vi "QR二维码生成器.vi"(6 "保存按钮":bool, 7 "输入文本":string="殷培\n2013年9月5日\nemail:yin-pei@qq.com", 8 "掩模图形":u16(ring) items=["000", "001", "010", "011", "100", "101", "110", "111"], 9 "版本":u16(ring)=1 items=["1"=1, "2"=2, "3"=3, "4"=4, "5"=5, "6"=6, "7"=7, "8"=8, "9"=9, "10"=10, "11"=11, "12"=12, "13"=13, "14"=14, "15"=15, "16"=16, "17"=17, "18"=18, "19"=19, "20"=20, "21"=21, "22"=22, "23"=23, "24"=24, "25"=25, "26"=26, "27"=27, "28"=28, "29"=29, "30"=30, "31"=31, "32"=32, "33"=33, "34"=34, "35"=35, "36"=36, "37"=37, "38"=38, "39"=39, "40"=40], 10 "纠错等级":u16(ring)=2 items=["L(7%)", "M(15%)", "Q(25%)", "H(30%)"], 11 "自动？":enum16{"禁止自适应版本", "自适应版本"}(ring)=enum."自适应版本") -> (3 "new picture":picture caption="新图片")   [LabVIEW 2011]
uses:
  <vilib>/Utility/miscctls.llb/LVBoundsTypeDef.ctl
panel:
  in  "添加logo":bool
  in  "停止":bool
  in  "backcolor":u32(colorbox)=16777215
  in  "color":u32(colorbox)
  # "QR二维码生成器"
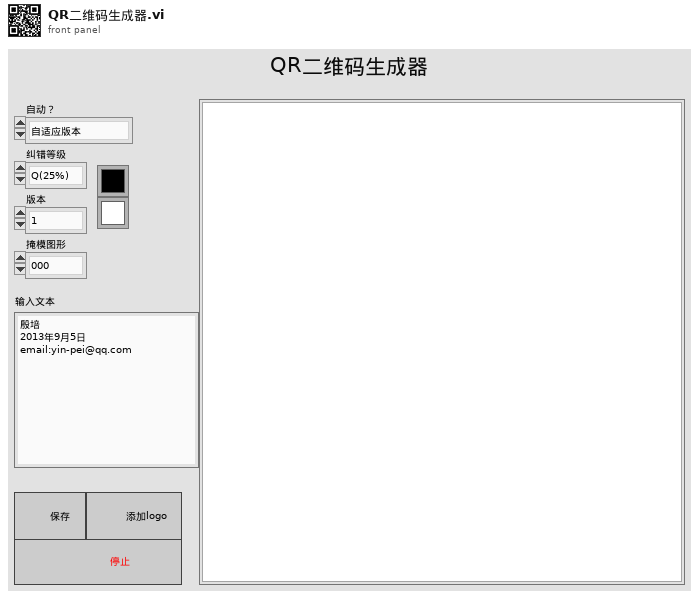
[diagram p1: front panel]
types:
  T1 = cluster{"left":i16, "top":i16, "right":i16, "bottom":i16}
  T2 = typedef "LVBoundsTypeDef.ctl" = cluster{"Width":u32, "Height":u32}
  T3 = typedef "imagedata.ctl" = cluster{"image type":i32, "image depth":i32, "image":u8[], "mask":u8[], "colors":u32[], "Rectangle":cluster{"left":i16, "top":i16, "right":i16, "bottom":i16}}
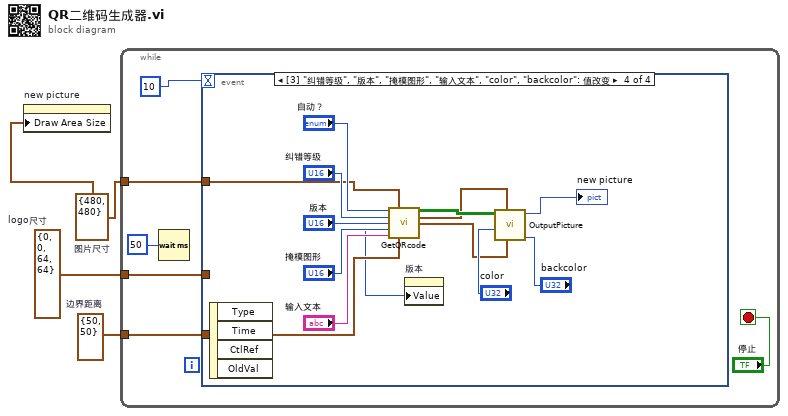
[diagram p0: block diagram]
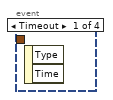
[diagram p2: hidden frame]
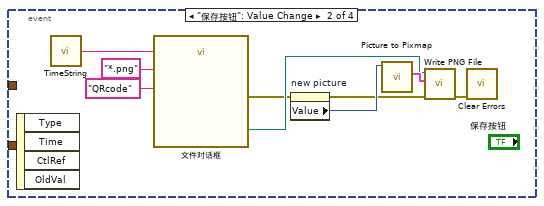
[diagram p3: hidden frame]
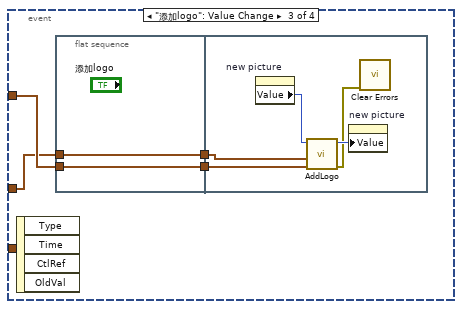
[diagram p4: hidden frame]
diagram:
  w1 = T1 {"left"=0, "top"=0, "right"=64, "bottom"=64}  # logo尺寸
  w2 = cluster{"x":i16, "y":i16} {"x"=50, "y"=50}  # 边界距离
  w3 = T2 {"Width"=480, "Height"=480}  # 图片尺寸
  n1 = property on="new picture" class="Pict"("Draw Area Size"=w3) -> ()  [unwired: 2 in, 2 out]
  n2 = while {
    tunnel: w3 -> [w6]
    tunnel: w2 -> [w5]
    tunnel: w1 -> [w4]
    stop <- "停止" stop-if-true
    n3 = Wait (ms)(milliseconds to wait=u32 50 ("等待时间（毫秒）")) -> ()  [unwired: 1 out]
    n4 = event shown="[3] \"纠错等级\", \"版本\", \"掩模图形\", \"输入文本\", \"color\", \"backcolor\": 值改变" {
      selector: _ -> [_ _ _ _]
      dyn-events: _ -> [_ _ _ _]
      timeout: 10 -> [_ _ _ _]
      tunnel: w6 -> [_ _ w22 w32]
      tunnel: w5 -> [_ _ _ w31]
      tunnel: w4 -> [_ _ w21 _]
      event Timeout {
        n5 = event-data() -> ()  [unwired: 1 in, 2 out]
      }
      event "保存按钮": Value Change {
        n6 = event-data() -> ()  [unwired: 1 in, 4 out]
        n7 = call "TimeString.vi"() -> ("时间字符串"=w12:string)
        n8 = call "文件对话框"("default name"=w12, "pattern (all files)"="*.png", "pattern label"="QRcode") -> ("selected path"=w14:path, "error out"=w13:errorcluster)  [unwired: 9 in, 2 out]
        n9 = property on="new picture" class="Pict"(error in=w13) -> (error out=w15:errorcluster, "Value"=w18:picture)  [unwired: 1 in, 1 out]
        n10 = call <vilib>:"Picture to Pixmap.vi"("picture"=w18) -> ("image data"=w17:T3)  [unwired: 9 in, 1 out]
        n11 = call <vilib>:"Write PNG File.vi"("error in (no error)"=w15, "image data"=w17, "path to PNG file"=w14) -> ("error out"=w16:errorcluster)  [unwired: 7 in, 1 out]
        n12 = call <vilib>:"Clear Errors.vi"("error in (no error)"=w16) -> ()  [unwired: 6 in, 1 out]
      }
      event "添加logo": Value Change {
        n13 = event-data() -> ()  [unwired: 1 in, 4 out]
        n14 = flat-sequence {
          tunnel: w21 -> [w23]
          tunnel: w22 -> [w24]
          tunnel: [w24] -> w20
          tunnel: [w23] -> w19
          tunnel: w20 -> [w27]
          tunnel: w19 -> [w26]
          frame #0 {
          }
          frame #1 {
            n15 = property on="new picture" class="Pict"() -> ("Value"=w29:picture)  [unwired: 2 in, 2 out]
            n16 = call "AddLogo.vi"("图片尺寸"=w27, "logo尺寸"=w26, "图片输入"=w29) -> ("error out"=w25:errorcluster, "图片输出"=w28:picture)  [unwired: 7 in]
            n17 = property on="new picture" class="Pict"("Value"=w28) -> ()  [unwired: 2 in, 2 out]
            n18 = call <vilib>:"Clear Errors.vi"("error in (no error)"=w25) -> ()  [unwired: 6 in, 1 out]
          }
        }
      }
      event "纠错等级", "版本", "掩模图形", "输入文本", "color", "backcolor": Value Change {
        n19 = event-data() -> ()  [unwired: 1 in, 4 out]
        n20 = call "GetQRcode.vi"("自动？"="自动？", "图片尺寸"=w32, "纠错等级"="纠错等级", "版本"="版本", "掩模图形"="掩模图形", "输入文本"="输入文本", "边界距离"=w31) -> ("二维码"=w35:bool[][], "显示起点"=w34:cluster{dbl, dbl}, "像素大小"=w33:cluster{dbl, dbl}, "扩展版本"=w30:i32)  [unwired: 5 in]
        n21 = property on="版本" class="Ring (严格)"("Value"=w30) -> ()  [unwired: 2 in, 2 out]
        n22 = call "OutputPicture.vi"("像素大小"=w33, "显示起点"=w34, "backcolor"="backcolor", "color"="color", "二维码"=w35) -> ("new picture"=→"new picture":picture)  [unwired: 6 in]
      }
    }
  }
